vi "SendAck.vi"(8 "error in (no error)":errorcluster, 9 "Ack":refnum<notifier>, 10 "Variant":variant) -> (0 "error out":errorcluster)   [LabVIEW 2017, in "Communication.lvlib"]
uses:
  Communication.lvlib
  MsgAck.ctl
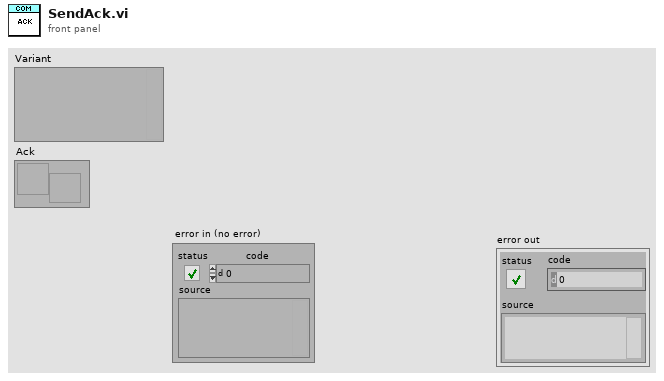
[diagram p1: front panel]
types:
  T1 = typedef "Communication.lvlib/MsgAck.ctl" = cluster{"Variant":variant, "error ":errorcluster}
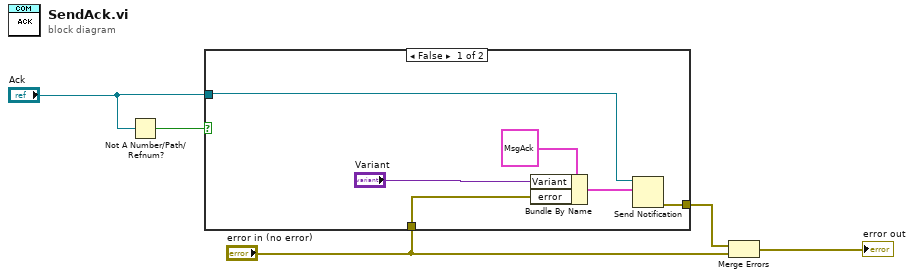
[diagram p0: block diagram]
diagram:
  n1 = Not A Number/Path/Refnum?(number/path/refnum="Ack") -> (NaN/Path/Refnum?=w4:bool)
  n2 = case shown="False" w4 {
    tunnel: "error in (no error)" -> [w11 w12]
    tunnel: "Ack" -> [w7 _]
    tunnel: [w6 w12] -> w1
    frame False {
      n3 = Bundle By Name(cluster=T1 {"Variant"=variant, "error "={"status"=FALSE, "code"=0, "source"=""}} ("notification"), "Variant"="Variant", "error"=w11) -> (w8:T1)
      n4 = Send Notification(notification=w8, notifier=w7) -> (error out=w6:errorcluster)  [unwired: 1 in, 1 out]
    }
    frame True {
    }
  }
  n5 = Merge Errors(w1, "error in (no error)") -> (→"error out":errorcluster)
